vi "RNG In Range.vi"(9 "llimit 2 (1)":dbl=1.0 format="%#_13g", 11 "limit 1 (0)":dbl) -> (3 "number":dbl)   [LabVIEW 2019, in "ACSVcontrol-driver.lvlib"]
uses:
  ACSVcontrol-driver.lvlib
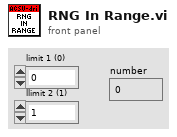
[diagram p1: front panel]
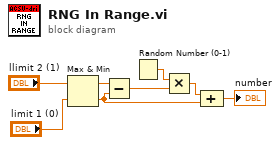
[diagram p0: block diagram]
diagram:
  n1 = Max & Min(x="llimit 2 (1)", y="limit 1 (0)") -> (max(x,y)=w1:dbl, min(x,y)=w2:dbl)
  n2 = Subtract(x=w1, y=w2) -> (x-y=w5:dbl)
  n3 = Random Number (0-1)() -> (number: 0 to 1=w8:dbl)
  n4 = Multiply(x=w8, y=w5) -> (x*y=w7:dbl)
  n5 = Compound Arithmetic op=ADD(w7, w2) -> (→"number":dbl)
